vi "__Alicat SD_ReadConfig.vi"(6 "Nodos":i32=4, 8 "error in":errorcluster, 10 "aDispositivos":T1=[["A", "NO", "aM0000013", "Air", "100", "ln/mn", "0.1", "0.11"], ["B", "NO", "aM0000014", "Air", "100", "ln/mn", "0.2", "0.22"], ["C", "NO", "aM0000015", "Air", "100", "ln/mn", "0.3", "0.33"], ["D", "NO", "aM0000016", "Air", "500", "ln/mn", "0.4", "0.44"]] caption="Alicats in", 11 "COMMS":T2={"Bronk mfc1"="ASRL6::INSTR", "Brk1"=FALSE, "Bronk mfc2"="ASRL6::INSTR", "Brk2"=FALSE, "Bronk mfc3"="ASRL6::INSTR", "Brk3"=FALSE, "Bronk mfc4"="ASRL6::INSTR", "Brk4"=FALSE, "Bronk mfm1"="ASRL6::INSTR", "Brkm"=FALSE, "Alicats"="ASRL6::INSTR", "Alic"=FALSE, "eVal4vias"="ASRL6::INSTR", "ev4v"=FALSE, "eVal3vias"="ASRL6::INSTR", "ev3v"=FALSE, "Cell GAS"="ASRL6::INSTR", "cgas"=FALSE, "Cell H2S"="ASRL6::INSTR", "ch2s"=FALSE}) -> (0 "error out":errorcluster, 1 "ParsedReadingArray":T3[](array[typedef]) {"SetPoint" format="%.2f"; "Mass" format="%.2f"; "Volumetric" format="%.2f"; "Temperature" format="%.2f"; "Pressure" format="%.2f"}, 2 "aDispositivos 2":T1=[["A", "NO", "aM0000013", "Air", "100", "ln/mn", "0.1", "0.11"], ["B", "NO", "aM0000014", "Air", "100", "ln/mn", "0.2", "0.22"], ["C", "NO", "aM0000015", "Air", "100", "ln/mn", "0.3", "0.33"], ["D", "NO", "aM0000016", "Air", "500", "ln/mn", "0.4", "0.44"]] caption="Alicats out")   [LabVIEW 2017]
uses:
  __Alicat SD_ReadingCluster.ctl
  KISSIA_COMUNICACIONES.ctl
  SERIAL BRONKHORST/__s_TablaBronkhorst.ctl
  __Alicat SD_Hardware_Module.ctl
  KISSIA_GLOBALES.vi
panel:
  out "ID(NODO)":string[](array[string])
  out "CONECTADO":bool[](array[boolean])
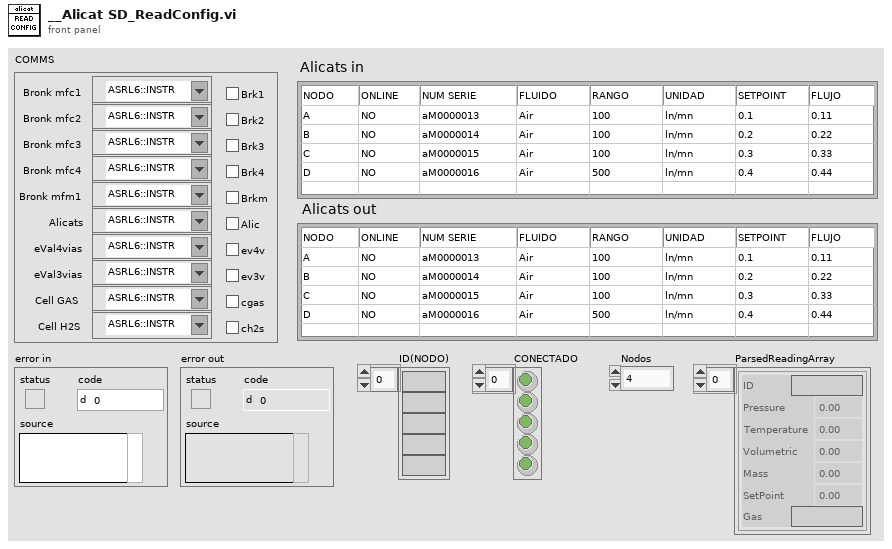
[diagram p1: front panel]
types:
  T1 = typedef "__s_TablaBronkhorst.ctl" = string[][]
  T2 = typedef "KISSIA_COMUNICACIONES.ctl" = cluster{"Bronk mfc1":refnum<visa-resource-name>, "Brk1":bool, "Bronk mfc2":refnum<visa-resource-name>, "Brk2":bool, "Bronk mfc3":refnum<visa-resource-name>, "Brk3":bool, "Bronk mfc4":refnum<visa-resource-name>, "Brk4":bool, "Bronk mfm1":refnum<visa-resource-name>, "Brkm":bool, "Alicats":refnum<visa-resource-name>, "Alic":bool, "eVal4vias":refnum<visa-resource-name>, "ev4v":bool, "eVal3vias":refnum<visa-resource-name>, "ev3v":bool, "Cell GAS":refnum<visa-resource-name>, "cgas":bool, "Cell H2S":refnum<visa-resource-name>, "ch2s":bool}
  T3 = typedef "__Alicat SD_ReadingCluster.ctl" = cluster{"ID":string, "Pressure":sgl, "Temperature":sgl, "Volumetric":sgl, "Mass":sgl, "SetPoint":sgl, "Gas":string}
  T4 = typedef "__Alicat SD_Hardware_Module.ctl" = enum16{"Initialize", "Send Setpoint", "Read Data", "Change Address", "Shutdown"}
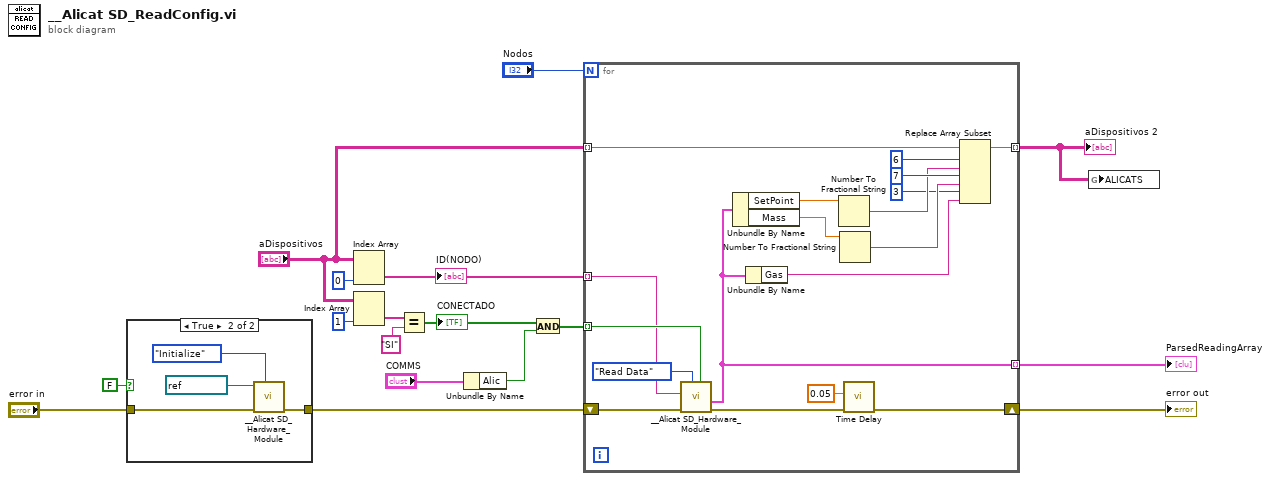
[diagram p0: block diagram]
diagram:
  n1 = case shown="True" FALSE {
    tunnel: "error in" -> [w18 w22]
    tunnel: [w18 w21] -> w10
    frame False {
    }
    frame True {
      n2 = call "__Alicat SD_Hardware_Module.vi"("Command"=__Alicat_SD_Hardware_Module."Initialize", "error in (no error)"=w22, "VISA resource name"=refnum<visa-resource-name> "COM9") -> ("error out"=w21:errorcluster)  [unwired: 5 in, 3 out]
    }
  }
  n3 = Index Array(array="aDispositivos", index (col)=0 ("disabled index (col)")) -> (element=w13:string[])  [unwired: 1 in]
  "ID(NODO)" <- w13
  n4 = Index Array(array="aDispositivos", index (col)=1 ("disabled index (col)")) -> (element=w16:string[])  [unwired: 1 in]
  n5 = Equal?(x=w16, y="SI") -> (x = y?=w7:bool[])
  "CONECTADO" <- w7
  n6 = Unbundle By Name("COMMS") -> ("Alic"=w6:bool)
  n7 = And(x=w7, y=w6) -> (x .and. y?=w8:bool[])
  n8 = for {
    N: "Nodos" -> [_]
    shift-right: [w34] -> w12
    shift-left: w10 -> [w40]
    tunnel: w8 -> [w38] mode=indexing
    tunnel: w13 -> [w37] mode=indexing
    tunnel: [w24] -> w5 mode=indexing
    tunnel: "aDispositivos" -> [w29] mode=indexing
    tunnel: [w28] -> w1 mode=indexing
    n9 = call "__Alicat SD_Hardware_Module.vi"("Used ?"=w38, "Command"=__Alicat_SD_Hardware_Module."Read Data", "error in (no error)"=w40, "Address"=w37) -> ("error out"=w35:errorcluster, "ParsedReading"=w24:T3)  [unwired: 4 in, 2 out]
    n10 = Unbundle By Name(w24) -> ("SetPoint"=w33:sgl, "Mass"=w32:sgl)
    n11 = Unbundle By Name(w24) -> ("Gas"=w23:string)
    n12 = Number To Fractional String(number=w33) -> (F-format string=w27:string)  [unwired: 3 in]
    n13 = Number To Fractional String(number=w32) -> (F-format string=w26:string)  [unwired: 3 in]
    n14 = call "Time Delay"("error in (no error)"=w35, "Delay Time (s)"=0.05) -> ("error out"=w34:errorcluster)  [unwired: 9 in]
    n15 = Replace Array Subset(array=w29, new element #1=w27, index #1=6 ("index"), new element #2=w26, index #2=7 ("index"), new element #3=w23, index #3=3 ("index")) -> (w28:string[])
  }
  "error out" <- w12
  "ParsedReadingArray" <- w5
  "aDispositivos 2" <- w1
  n16 = global write "KISSIA_GLOBALES.vi" "ALICATS"(w1) -> ()
